vi "Python@GetVariable(Session)__Parameter.vi"(1 "ParamterIn":string) -> (0 "ParamterOut":string)   [LabVIEW 2020]
panel:
  in  "Session":string(combo)
  in  "ARCOSName":string(combo) caption="ARCOSName="
  in  "Section":string(combo)
  in  "PythonVariable":string(combo)
  in  "Confirm":bool
  # "Python@GetVariable(Session) $Session,$PythonVariable(,$section,ARCOSName=)"
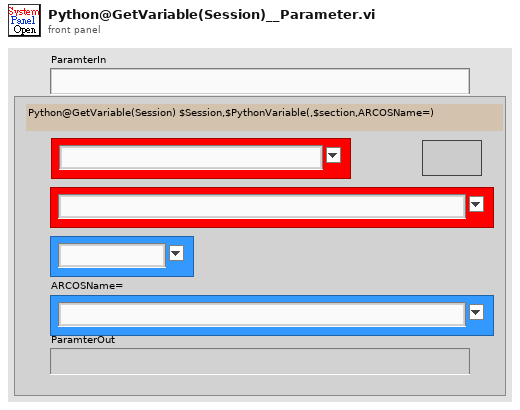
[diagram p1: front panel]
types:
  T1 = enum16{"Get", "Init", "Set", "Delete", "GetElement", "Inc", "Dec", "ReName"}
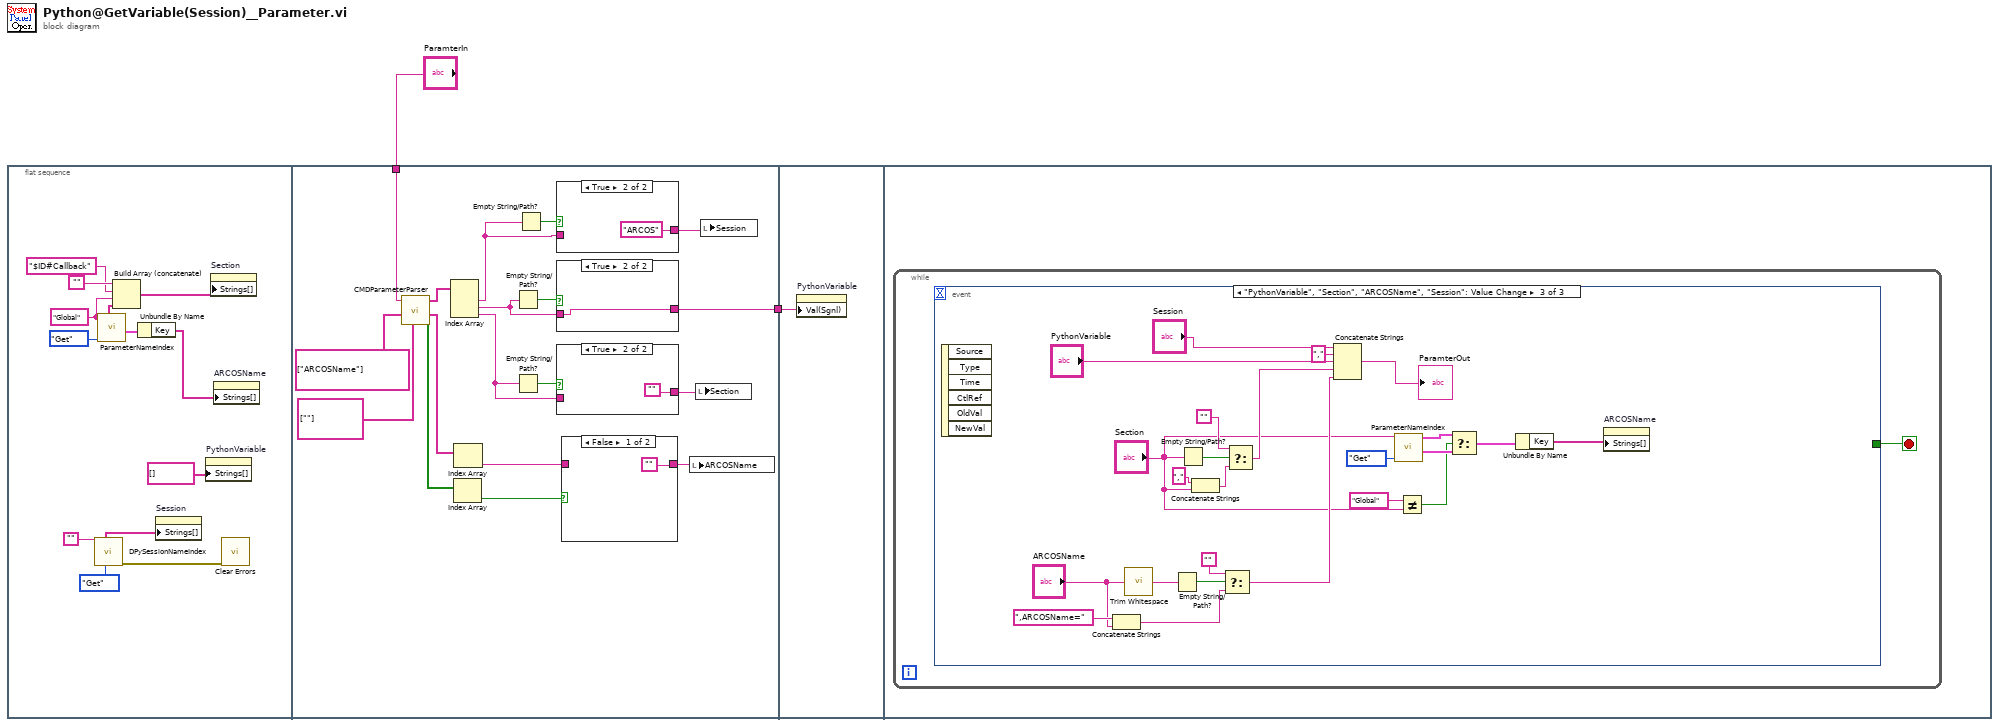
[diagram p0: block diagram]
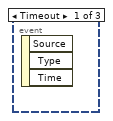
[diagram p6: hidden frame]
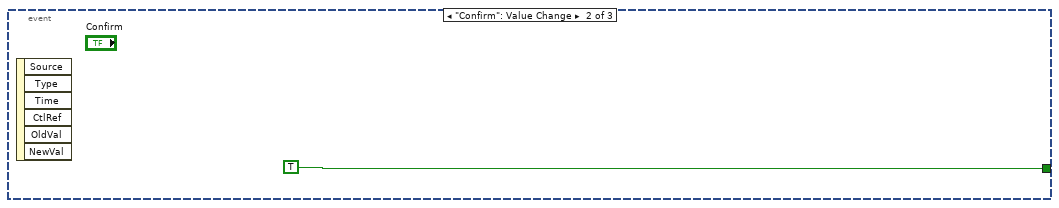
[diagram p7: hidden frame]
diagram:
  n1 = flat-sequence {
    tunnel: "ParamterIn" -> [w27]
    tunnel: [w32] -> w1
    tunnel: w1 -> [w42]
    frame #0 {
      w11 = "Global" ("VariableSection")
      n2 = call "DPySessionNameIndex.vi"("OP"=enum16{"Init", "Get", "Set"}."Get", "SessionIn"="") -> ("error out"=w3:errorcluster, "DPythonSessionNameS"=w4:string[])  [unwired: 6 in, 2 out]
      n3 = call "ParameterNameIndex.vi"("OP"=T1."Get", "VariableSection"=w11) -> ("GlobalKeyValue"=w15:cluster{"Key":string[], "Value":string[]}, "SectionList"=w12:string[])  [unwired: 3 in, 5 out]
      n4 = Build Array (concatenate)("", "$ID#Callback" ("VariableSection"), w11, w12) -> (w10:string[])
      n5 = Unbundle By Name(w15) -> ("Key"=w8:string[])
      n6 = property on="Session" class="CmbBox"("Strings[]"=w4) -> ()  [unwired: 2 in, 2 out]
      n7 = property on="PythonVariable" class="CmbBox"("Strings[]"=string[] [] ("Strings []")) -> ()  [unwired: 2 in, 2 out]
      n8 = property on="Section" class="CmbBox"("Strings[]"=w10) -> ()  [unwired: 2 in, 2 out]
      n9 = property on="ARCOSName" class="CmbBox"("Strings[]"=w8) -> ()  [unwired: 2 in, 2 out]
      n10 = call <vilib>:"Clear Errors.vi"("error in (no error)"=w3) -> ()  [unwired: 5 in, 2 out]
    }
    frame #1 {
      n11 = call "CMDParameterParser.vi"("DeafultValues"=string[] [""], "RequiredKeys"=string[] ["ARCOSName"], "CMDParameter"=w27) -> ("KeyFind?"=w22:bool[], "KeyValues"=w23:string[], "Input"=w26:string[])  [unwired: 6 in]
      n12 = Index Array(array=w26) -> (element #1=w17:string, element #2=w31:string, element #3=w28:string)  [unwired: 3 in]
      n13 = Index Array(array=w22) -> (element=w21:bool)  [unwired: 1 in]
      n14 = Index Array(array=w23) -> (element=w20:string)  [unwired: 1 in]
      n15 = Empty String/Path?(string/path=w31) -> (empty?=w33:bool)
      n16 = Empty String/Path?(string/path=w28) -> (empty?=w30:bool)
      n17 = Empty String/Path?(string/path=w17) -> (empty?=w18:bool)
      n18 = case shown="True" w18 {
        tunnel: w17 -> [w34 _]
        tunnel: [w34 "ARCOS"] -> w16
        frame False {
        }
        frame True {
        }
      }
      n19 = case shown="True" w33 {
        tunnel: w31 -> [w40 w41]
        tunnel: [w40 w41] -> w32
        frame False {
        }
        frame True {
        }
      }
      n20 = case shown="True" w30 {
        tunnel: w28 -> [w38 _]
        tunnel: [w38 ""] -> w29
        frame False {
        }
        frame True {
        }
      }
      n21 = case shown="False" w21 {
        tunnel: w20 -> [_ w37]
        tunnel: ["" w37] -> w19
        frame False {
        }
        frame True {
        }
      }
      n22 = local write "ARCOSName"(w19) -> ()
      n23 = local write "Section"(w29) -> ()
      n24 = local write "Session"(w16) -> ()
    }
    frame #2 {
      n25 = property on="PythonVariable" class="CmbBox"("Val(Sgnl)"=w42) -> ()  [unwired: 2 in, 2 out]
    }
    frame #3 {
      n26 = while {
        stop <- w43 stop-if-true
        n27 = event shown="[2] \"PythonVariable\", \"Section\", \"ARCOSName\", \"Session\": Value Change" {
          selector: _ -> [_ _ _]
          dyn-events: _ -> [_ _ _]
          timeout: _ -> [_ _ _]
          tunnel: [_ TRUE _] -> w43
          event Timeout {
            n28 = event-data() -> ()  [unwired: 1 in, 3 out]
          }
          event "Confirm": Value Change {
            n29 = event-data() -> ()  [unwired: 1 in, 6 out]
          }
          event "PythonVariable", "Section", "ARCOSName", "Session": Value Change {
            n30 = event-data() -> ()  [unwired: 1 in, 6 out]
            n31 = Concatenate Strings(",ARCOSName=" ("string"), "ARCOSName") -> (w54:string)
            n32 = call <vilib>:"Trim Whitespace.vi"("string"="ARCOSName") -> ("trimmed string"=w57:string)  [unwired: 1 in]
            n33 = Empty String/Path?(string/path=w57) -> (empty?=w56:bool)
            n34 = Empty String/Path?(string/path="Section") -> (empty?=w64:bool)
            n35 = Concatenate Strings("," ("string"), "Section") -> (w65:string)
            n36 = Select(t="", s=w56, f=w54) -> (s? t:f=w53:string)
            n37 = Select(t="", s=w64, f=w65) -> (s? t:f=w62:string)
            n38 = Concatenate Strings("Session", "," ("string"), "PythonVariable", w62, w53) -> (→"ParamterOut":string)
            n39 = call "ParameterNameIndex.vi"("OP"=T1."Get", "VariableSection"="Section") -> ("GlobalKeyValue"=w51:cluster{"Key":string[], "Value":string[]}, "SectionKeyValue"=w52:cluster{"Key":string[], "Value":string[]})  [unwired: 3 in, 5 out]
            n40 = Not Equal?(x="Global", y="Section") -> (x != y?=w47:bool)
            n41 = Select(t=w52, s=w47, f=w51) -> (s? t:f=w50:cluster{"Key":string[], "Value":string[]})
            n42 = Unbundle By Name(w50) -> ("Key"=w60:string[])
            n43 = property on="ARCOSName" class="CmbBox"("Strings[]"=w60) -> ()  [unwired: 2 in, 2 out]
          }
        }
      }
    }
  }
